vi "Get configuration chain.vi"(8 "error in (no error)":errorcluster, 11 "CascadeBase in":refnum<class "Cascade.lvclass">) -> (0 "error out":errorcluster, 1 "class name":string[](array[string]), 2 "configuration chain":variant[](array[variant]), 3 "CascadeBase out":refnum<class "Cascade.lvclass">)   [LabVIEW 2012, in "Cascade.lvclass"]
doc: "Returns an array of variants containing the configuration clusters of each class in the inheritance chain (lowest child class first), together with an array of all class names in the inheritance chain.\n\nFor classes without configuration cluster, the configuration chain contains empty variants."
uses:
  Cascade.lvclass
  <vilib>/Distrio/Murmex/Murmex/Murmex.lvclass
  Cascade.lvclass/Cascade.ctl
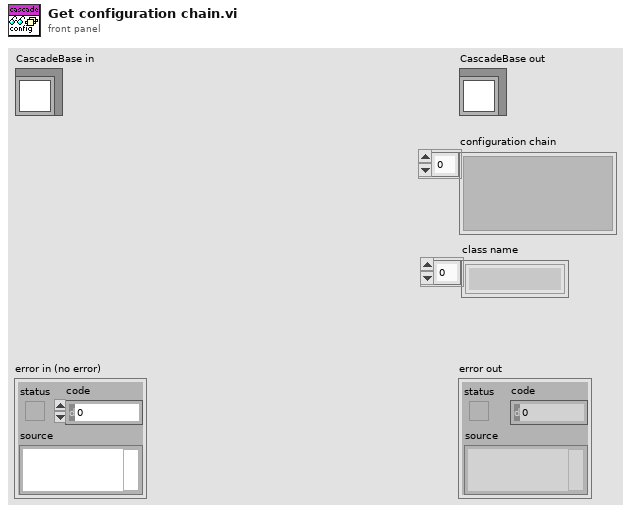
[diagram p1: front panel]
types:
  T1 = typedef "Cascade.lvclass/configuration.ctl" = cluster{"Timing mode":T2, "Trigger Edge":T3, "Temperature":dbl, "Number of frames":u32, "LUT":path, "stage component":string, "Background image":path, "Accumulations":u32, "Gain mode":T4, "Acquire flag":T5, "micron equivalent of pixel":dbl[unit], "max x pixel displacement":dbl, "min x pixel displacement":dbl, "max pixel discrepancy":dbl, "max y pixel displacement":dbl, "min y pixel displacement":dbl, "brightness threshold":sgl}
  T2 = typedef "Cascade.lvclass/timing mode.ctl" = u32
  T3 = typedef "Cascade.lvclass/Trigger edge.ctl" = u32
  T4 = typedef "Cascade.lvclass/gain mode.ctl" = u32
  T5 = typedef "Cascade.lvclass/acquire flag.ctl" = u32
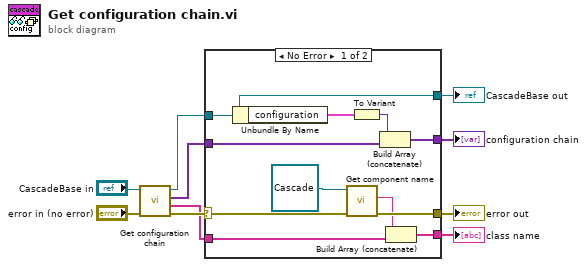
[diagram p0: block diagram]
diagram:
  n1 = call-parent "Get configuration chain.vi"("error in (no error)"="error in (no error)", "MurmexBase in"="CascadeBase in") -> ("error out"=w8:errorcluster, "class name"=w6:string[], "configuration chain"=w3:variant[], "MurmexBase out"=w4:refnum<class "Cascade.lvclass">)  [unwired: 6 in]
  n2 = case shown="No Error" w8 {
    selector: w8 -> [w21 w22]
    tunnel: [w20 w22] -> w7
    tunnel: w6 -> [w17 _]
    tunnel: [w16 _] -> w5
    tunnel: w4 -> [w11 w23]
    tunnel: w3 -> [w13 _]
    tunnel: [w12 _] -> w2
    tunnel: [w11 w23] -> w1
    frame No Error {
      n3 = Unbundle By Name(w11) -> ("configuration"=w15:T1)
      n4 = call <vilib>:"Get component name.vi"("error in (no error)"=w21, "Murmex in"=refnum<class "Cascade.lvclass"> refnum ("Cascade.lvclass")) -> ("error out"=w20:errorcluster, "component name"=w18:string)  [unwired: 7 in, 1 out]
      n5 = To Variant(anything=w15) -> (Variant=w14:variant)
      n6 = Build Array (concatenate)(w14, w13) -> (w12:variant[])
      n7 = Build Array (concatenate)(w18, w17) -> (w16:string[])
    }
    frame Error {
    }
  }
  "error out" <- w7
  "CascadeBase out" <- w1
  "configuration chain" <- w2
  "class name" <- w5
